vi "read_comm_definition.vi"(8 "error in (no error)":errorcluster, 11 "file path (dialog if empty)":path) -> (0 "error out":errorcluster, 2 "Comm variable definitions":T1[](array[typedef]) {"Cluster"."Mode" items=["None", "MODBUS", "HART", "Profibus DP", "Profibus PA", "Fieldbus", "DeviceNET"]}, 3 "all rows":string[][](array[string]))   [LabVIEW 2016]
uses:
  Typedef/comm_variable_definition.ctl
  Typedef/Comm_mode_and_address_type.ctl
  Typedef/Comm_mode_type_combo.ctl
  <vilib>/Utility/file.llb/Read From Spreadsheet File (string).vi
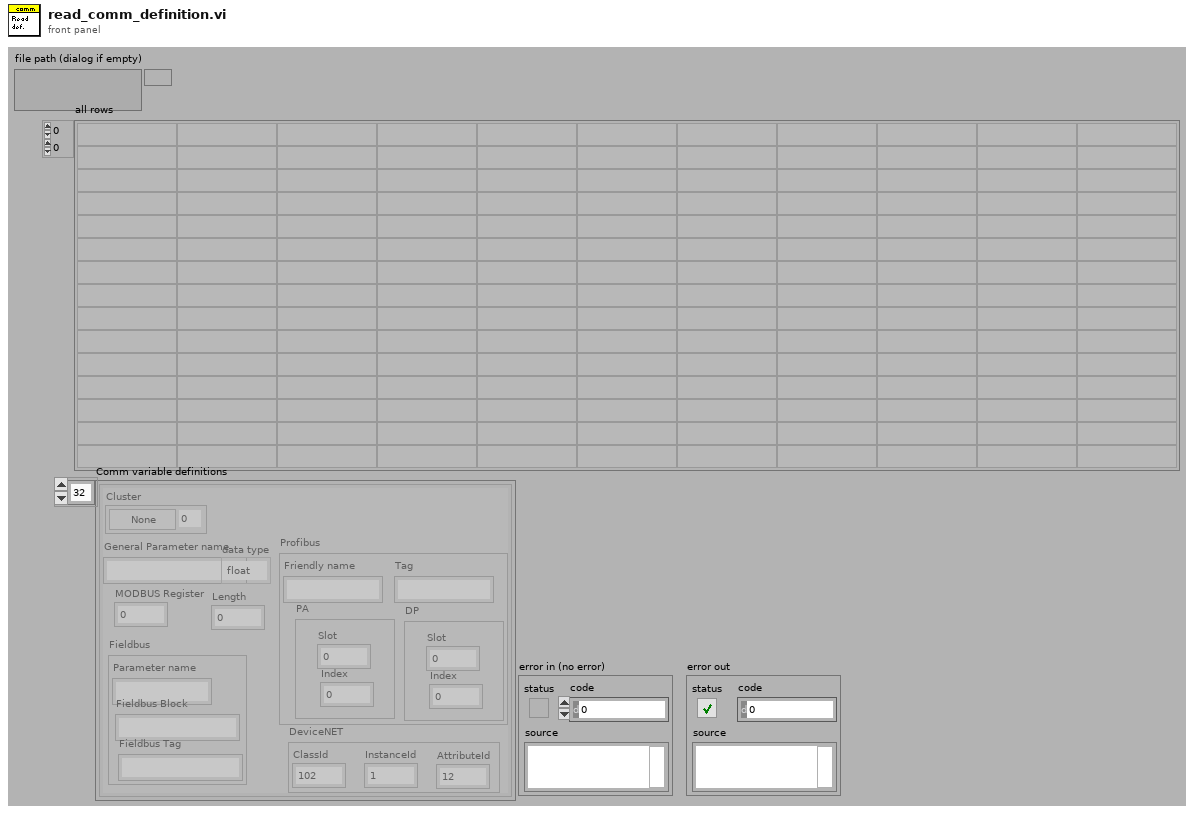
[diagram p1: front panel]
types:
  T1 = typedef "comm_variable_definition.ctl" = cluster{"General Parameter name":string, "MODBUS Register":i32, "Profibus":cluster{"Friendly name":string, "PA":cluster{"Slot":i32, "Index":i32}, "DP":cluster{"Slot":i32, "Index":i32}, "Tag":string}, "Fieldbus":cluster{"Parameter name":string, "Fieldbus Block":string, "Fieldbus Tag":string}, "data type":enum16{"float", "UINT", "UINT32", "STRING"}, "DeviceNET":cluster{"ClassId":u16, "InstanceId":u16, "AttributeId":u8}, "Cluster":T2, "Length":i32}
  T2 = typedef "Comm_mode_and_address_type.ctl" = cluster{"address":i32, "Mode":T3}
  T3 = typedef "Comm_mode_type_combo.ctl" = u16
  T4 = cluster{"Friendly name":string, "PA":cluster{"Slot":i32, "Index":i32}, "DP":cluster{"Slot":i32, "Index":i32}, "Tag":string}
  T5 = cluster{"String":string, "String":string, "String":string}
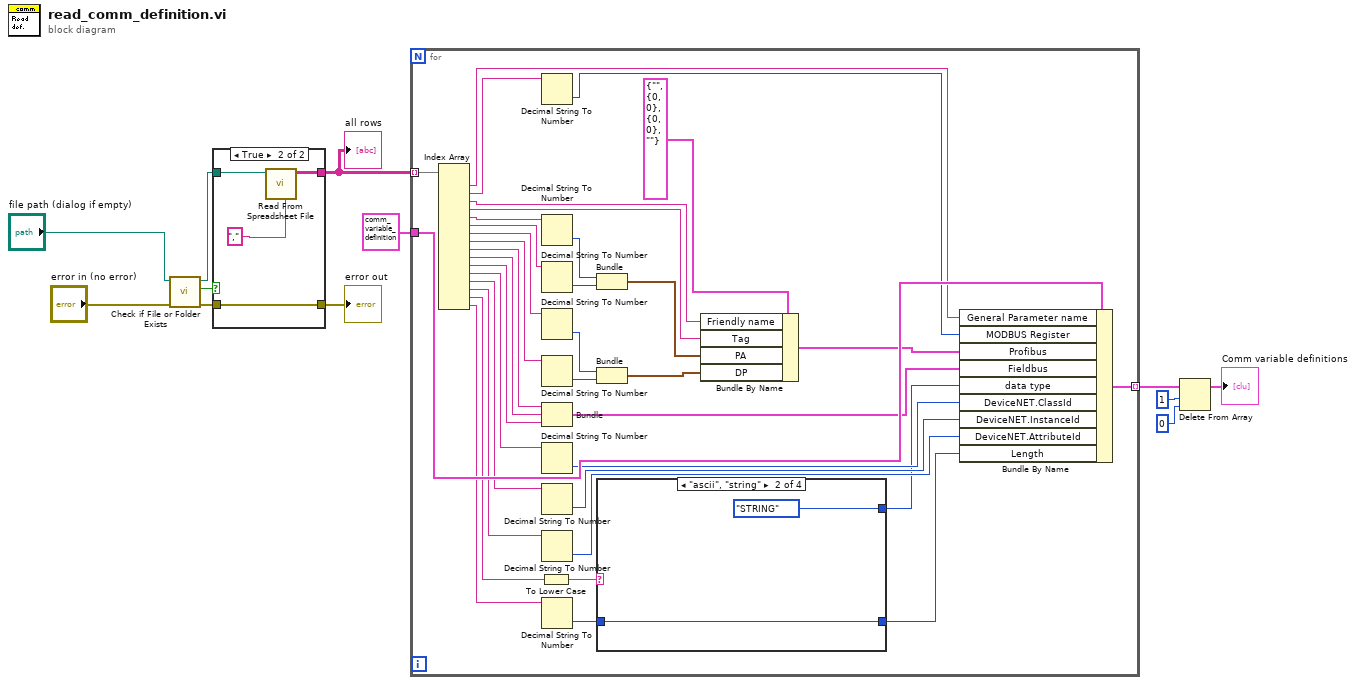
[diagram p0: block diagram]
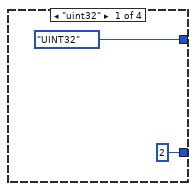
[diagram p3: hidden frame]
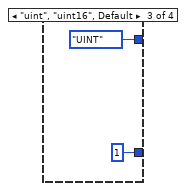
[diagram p4: hidden frame]
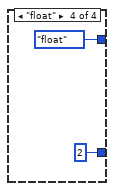
[diagram p5: hidden frame]
diagram:
  n1 = call <vilib>:"Check if File or Folder Exists.vi"("error in (no error)"="error in (no error)", "path"="file path (dialog if empty)") -> ("error out"=w3:errorcluster, "file or folder exists?"=w4:bool, "dup path"=w5:path)  [unwired: 7 in]
  n2 = case shown="True" w4 {
    tunnel: w5 -> [_ w17]
    tunnel: [_ w15] -> w11
    tunnel: w3 -> [w13 w14]
    tunnel: [w13 w14] -> w2
    frame False {
    }
    frame True {
      n3 = call-poly <vilib>:"Read From Spreadsheet File.vi"("delimiter (\\t)"="," ("delimiter (\\t)"), "file path (dialog if empty)"=w17) -> ("all rows"=w15:string[][])  [unwired: 5 in, 4 out]
    }
  }
  "all rows" <- w11
  "error out" <- w2
  n4 = for {
    tunnel: w11 -> [w52] mode=indexing
    tunnel: T1 {"General Parameter name"="", "MODBUS Register"=0, "Profibus"={"Friendly name"="", "PA"={"Slot"=0, "Index"=0}, "DP"={"Slot"=0, "Index"=0}, "Tag"=""}, "Fieldbus"={"Parameter name"="", "Fieldbus Block"="", "Fieldbus Tag"=""}, "data type"=enum."float", "DeviceNET"={"ClassId"=0, "InstanceId"=0, "AttributeId"=0}, "Cluster"={"address"=0, "Mode"=0}, "Length"=0} ("Comm definition type") -> [w53]
    tunnel: [w50] -> w9 mode=indexing
    n5 = Index Array(array=w52) -> (element #1=w51:string, element #2=w49:string, element #3=w47:string, element #4=w45:string, element #5=w44:string, element #6=w43:string, element #7=w38:string, element #8=w37:string, element #9=w33:string, element #10=w32:string, element #11=w30:string, element #12=w26:string, element #13=w25:string, element #14=w24:string, element #15=w23:string, element #16=w20:string)  [unwired: 16 in]
    n6 = To Lower Case(string=w23) -> (all lower case string=w21:string)
    n7 = Decimal String To Number(string=w49) -> (number=w48:i32)  [unwired: 2 in, 1 out]
    n8 = Decimal String To Number(string=w44) -> (number=w42:i32)  [unwired: 2 in, 1 out]
    n9 = Decimal String To Number(string=w43) -> (number=w41:i32)  [unwired: 2 in, 1 out]
    n10 = Decimal String To Number(string=w38) -> (number=w36:i32)  [unwired: 2 in, 1 out]
    n11 = Decimal String To Number(string=w37) -> (number=w39:i32)  [unwired: 2 in, 1 out]
    n12 = Bundle("String"=w33, "String"=w32, "String"=w30) -> (w31:T5)  [unwired: 1 in]
    n13 = Decimal String To Number(string=w26) -> (number=w29:i32)  [unwired: 2 in, 1 out]
    n14 = Decimal String To Number(string=w25) -> (number=w28:i32)  [unwired: 2 in, 1 out]
    n15 = Decimal String To Number(string=w24) -> (number=w27:i32)  [unwired: 2 in, 1 out]
    n16 = Decimal String To Number(string=w20) -> (number=w19:i32)  [unwired: 2 in, 1 out]
    n17 = Bundle(w42, w41) -> (w40:cluster{i32, i32})  [unwired: 1 in]
    n18 = Bundle(w36, w39) -> (w35:cluster{i32, i32})  [unwired: 1 in]
    n19 = case shown="\"ascii\", \"string\"" w21 {
      tunnel: [enum16{"float", "UINT", "UINT32", "STRING"}."UINT32" ("data type") enum16{"float", "UINT", "UINT32", "STRING"}."STRING" ("data type") enum16{"float", "UINT", "UINT32", "STRING"}."UINT" ("data type") enum16{"float", "UINT", "UINT32", "STRING"}."float" ("data type")] -> w22
      tunnel: w19 -> [_ w57 _ _]
      tunnel: [2 w57 1 2] -> w18
      frame "uint32" {
      }
      frame "ascii", "string" {
      }
      frame "uint", "uint16", Default {
      }
      frame "float" {
      }
    }
    n20 = Bundle By Name(cluster=T4 {"Friendly name"="", "PA"={"Slot"=0, "Index"=0}, "DP"={"Slot"=0, "Index"=0}, "Tag"=""} ("Profibus"), "Friendly name"=w47, "Tag"=w45, "PA"=w40, "DP"=w35) -> (w34:T4)
    n21 = Bundle By Name(cluster=w53, "General Parameter name"=w51, "MODBUS Register"=w48, "Profibus"=w34, "Fieldbus"=w31, "data type"=w22, "DeviceNET.ClassId"=w29, "DeviceNET.InstanceId"=w28, "DeviceNET.AttributeId"=w27, "Length"=w18) -> (w50:T1)
  }
  n22 = Delete From Array(array=w9, length=1, index=0) -> (array with subset deleted=→"Comm variable definitions":T1[])  [unwired: 1 out]
